vi "test Loopback_Acyclic Messages.vi"(8 "error in":errorcluster, 11 "TestCase in":refnum<class "Single Core Acyclic Loopback.lvclass">) -> (0 "error out":errorcluster, 3 "TestCase out":refnum<class "Single Core Acyclic Loopback.lvclass">)   [LabVIEW 2020, in "Single Core Acyclic Loopback.lvclass"]
uses:
  Single Core Acyclic Loopback.lvclass
  C:/Git/niveristand-custom-device-testing-tools/VeriStandTestCase/VeriStandTestCase.lvclass
  <vilib>/numeric/Random Number (Range) I64.vi
  <vilib>/numeric/sub_Random U32.vi
  <vilib>/NI VeriStand/Execution/Workspace/NI VeriStand - Set Multiple Channel Values.vi
  <vilib>/addons/_JKI Toolkits/VI Tester/TestCase.llb/TestCase.lvclass
  <vilib>/NI VeriStand/Execution/Workspace/NI_VS Workspace ExecutionAPI.lvlib
  C:/Program Files (x86)/National Instruments/LabVIEW 2020/vi.lib/addons/_JKI Toolkits/VI Tester/TestCase.llb/TestCase.lvclass
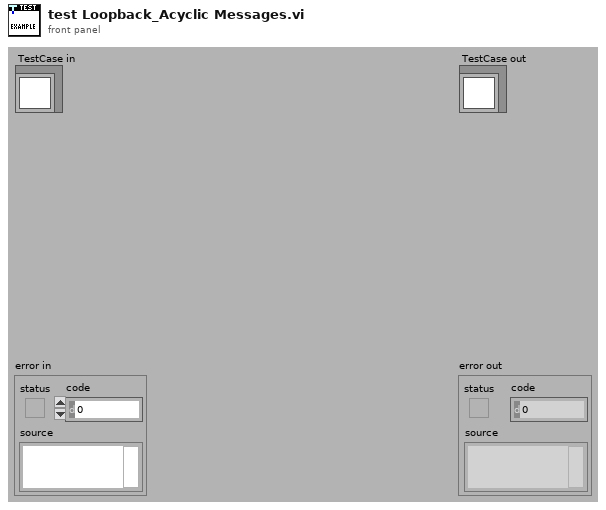
[diagram p1: front panel]
types:
  T1 = typedef "NI_VS Workspace ExecutionAPI.lvlib/WorkspaceAPI.ctl" = refnum<k24>
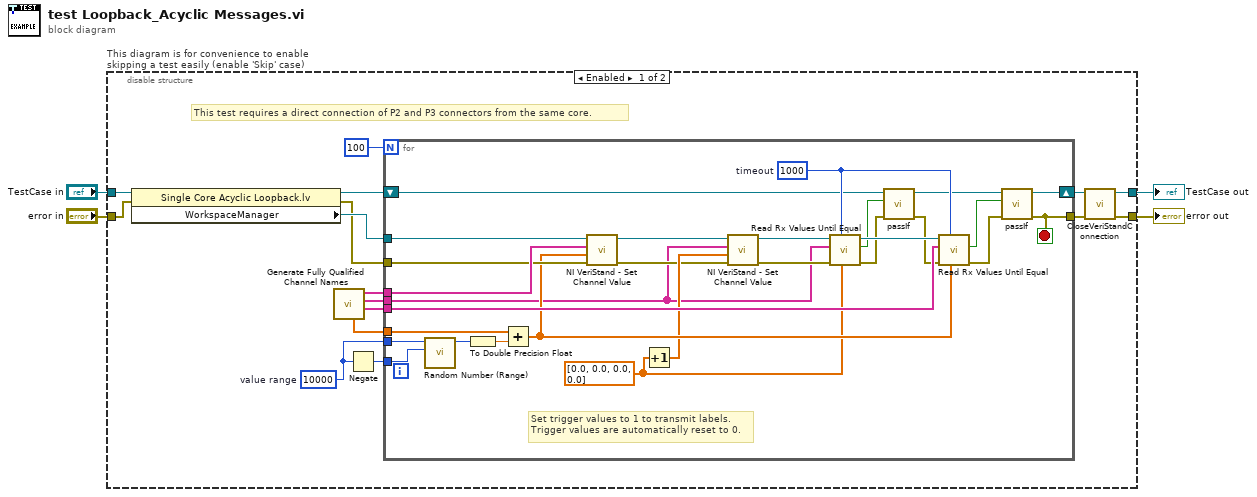
[diagram p0: block diagram]
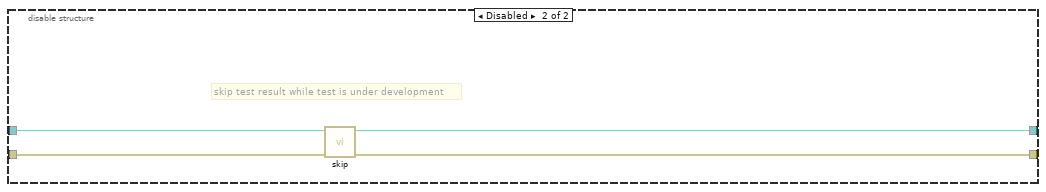
[diagram p2: hidden frame]
diagram:
  n1 = disable-structure "This diagram is for convenience to enable skipping a test easily (enable 'Skip' case)" shown="Enabled" {
    disable-tunnel: "TestCase in" -> [w20 w52]
    disable-tunnel: [w18 w50] -> w1
    disable-tunnel: [w17 w51] -> w3
    disable-tunnel: "error in" -> [w19 w49]
    frame Enabled {
      w15 = i64 10000  # value range
      # "This test requires a direct connection of P2 and P3 connectors from the same core."
      n2 = property class="Single Core Acyclic Loopback.lv"(reference=w20, error in=w19) -> (reference out=w9:refnum<class "Single Core Acyclic Loopback.lvclass">, error out=w11:errorcluster, "WorkspaceManager"=w12:T1)
      n3 = call "Generate Fully Qualified Channel Names.vi"() -> ("Rx channels"=w10:string[], "trigger channels"=w5:string[], "Tx channels"=w13:string[], "channel index"=w16:dbl[])  [unwired: 8 in]
      n4 = Negate(x=w15) -> (-x=w14:i64)
      n5 = for {
        N: 100 -> [_]
        tunnel: w16 -> [w46]
        tunnel: w15 -> [w45]
        tunnel: w14 -> [w44]
        tunnel: w13 -> [w43]
        tunnel: w12 -> [w42]
        tunnel: w11 -> [w41]
        tunnel: w10 -> [w40]
        shift-right: [w38] -> w8
        shift-left: w9 -> [w22]
        tunnel: [w36] -> w7
        tunnel: w5 -> [w28]
        stop <- w36 stop-if-true
        w27 = dbl[] [0.0, 0.0, 0.0, 0.0]
        w26 = 1000  # timeout
        # "Set trigger values to 1 to transmit labels. \nTrigger values are automatically reset to 0."
        n6 = call-poly <vilib>:"Random Number (Range).vi"("lower bound (-100)"=w44, "upper bound (100)"=w45) -> ("number"=w48:i64)  [unwired: 9 in]
        n7 = To Double Precision Float(number=w48) -> (double precision float=w47:dbl)
        n8 = Add(x=w46, y=w47) -> (x+y=w37:dbl[])
        n9 = call-poly <vilib>:"NI VeriStand - Set Channel Value.vi"("error in (no error)"=w41, "Values"=w37, "Channels"=w43, "WorkspaceManager in"=w42) -> ("error out"=w32:errorcluster, "WorkspaceManager out"=w33:T1)  [unwired: 6 in]
        n10 = Increment(x=w27) -> (x+1=w34:dbl[])
        n11 = call-poly <vilib>:"NI VeriStand - Set Channel Value.vi"("error in (no error)"=w32, "Values"=w34, "Channels"=w28, "WorkspaceManager in"=w33) -> ("error out"=w30:errorcluster, "WorkspaceManager out"=w31:T1)  [unwired: 6 in]
        n12 = call "Read Rx Values Until Equal.vi"("expected values"=w27, "timeout (1000 ms)"=w26, "error in"=w30, "Rx aliases"=w28, "workspace manager in"=w31) -> ("error out"=w23:errorcluster, "values equal expected"=w21:bool, "workspace manager out"=w29:T1)  [unwired: 4 in]
        n13 = call-dynamic "passIf.vi"("error in (no error)"=w23, "pass"=w21, "TestCase in"=w22) -> ("error out"=w24:errorcluster, "TestCase out"=w25:refnum<class "Single Core Acyclic Loopback.lvclass">)  [unwired: 7 in]
        n14 = call "Read Rx Values Until Equal.vi"("expected values"=w37, "timeout (1000 ms)"=w26, "error in"=w24, "Rx aliases"=w40, "workspace manager in"=w29) -> ("error out"=w39:errorcluster, "values equal expected"=w35:bool)  [unwired: 4 in, 1 out]
        n15 = call-dynamic "passIf.vi"("error in (no error)"=w39, "pass"=w35, "TestCase in"=w25) -> ("error out"=w36:errorcluster, "TestCase out"=w38:refnum<class "Single Core Acyclic Loopback.lvclass">)  [unwired: 7 in]
      }
      n16 = call-dynamic "CloseVeriStandConnection.vi"("error in (no error)"=w7, "VeriStand Test Case in"=w8) -> ("error out"=w17:errorcluster, "VeriStand Test Case out"=w18:refnum<class "Single Core Acyclic Loopback.lvclass">)  [unwired: 8 in]
    }
    frame Disabled {
      # "skip test result while test is under development"
      n17 = call <vilib>:"skip.vi"("error in (no error)"=w49, "TestCase in"=w52) -> ("error out"=w51:errorcluster, "TestCase out"=w50:refnum<class "Single Core Acyclic Loopback.lvclass">)  [unwired: 8 in]
    }
  }
  "error out" <- w3
  "TestCase out" <- w1
